vi "ICNC Get Sys Info.vi"(8 "error in (no error)":errorcluster caption="entrée d'erreur (pas d'erreur)", 10 "SysInfo":u32, 11 "SysInfoType":u32) -> (0 "error out":errorcluster caption="sortie d'erreur", 2 "SysInfo out":u32, 3 "function return":u32)   [LabVIEW 2012, in "ICNC2.lvlib"]
doc: "DWORD ICNC_GetSysInfo(DWORD SysInfoType,\n DWORD *SysInfo);"
uses:
  <userlib>/ICNC/ICNC2.lvlib
  <userlib>/ICNC/ICNC2.dll
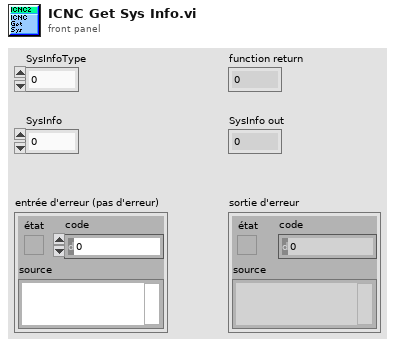
[diagram p1: front panel]
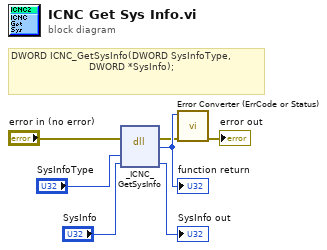
[diagram p0: block diagram]
diagram:
  # "DWORD ICNC_GetSysInfo(DWORD SysInfoType,\n                          DWORD *SysInfo);"
  n1 = dll-call lib="C:/Program Files (x86)/National Instruments/LabVIEW 2012/user.lib/ICNC/ICNC2.*" fn="_ICNC_GetSysInfo"(error in="error in (no error)", "SysInfoType"="SysInfoType", "SysInfo"="SysInfo") -> (error out=w2:errorcluster, w7:u32, "SysInfo"=→"SysInfo out":u32)  [unwired: 3 in, 1 out]
  "function return" <- w7
  n2 = call <userlib>:"Error Converter (ErrCode or Status).vi"("error in (no error)"=w2, "error code"=w7) -> ("error out"=→"error out":errorcluster)  [unwired: 9 in]
